vi "TiePie.Gen.Configure.vi"(8 "error in (no error)":errorcluster, 10 "Config":T1={"signal type (sine)"=1, "frequency"=0.0, "amplitude"=0.0, "offset"=0.0, "Enable"=FALSE} {"signal type (sine)" items=["sine"=1, "triangle"=2, "square"=4, "DC"=8, "noise"=16, "arbitrary"=32, "pulse"=64]}, 11 "GenHandle":T2) -> (0 "error out":errorcluster, 3 "GenHandle out":T2)   [LabVIEW 2013, in "LVTiePie.lvlib"]
uses:
  LVTiePie.lvlib
  TiePie.Gen.handle.ctl
  TiePie.Gen.CfgData.ctl
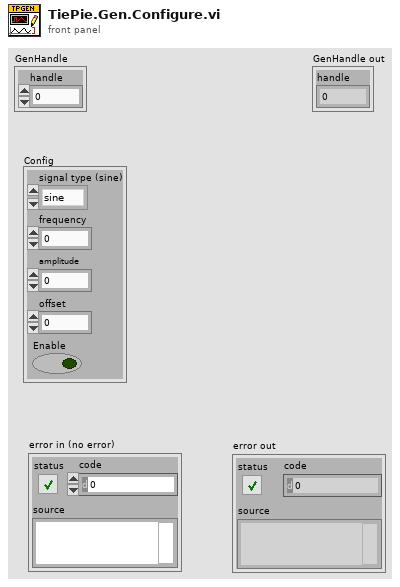
[diagram p1: front panel]
types:
  T1 = typedef "TiePie.Gen.CfgData.ctl" = cluster{"signal type (sine)":u32, "frequency":dbl, "amplitude":dbl, "offset":dbl, "Enable":bool}
  T2 = typedef "TiePie.Gen.handle.ctl" = cluster{"handle":u32}
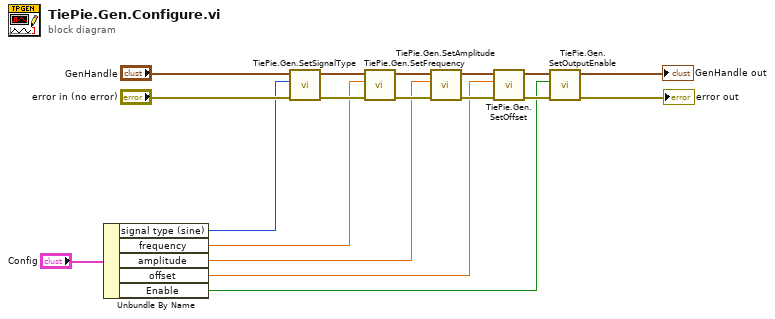
[diagram p0: block diagram]
diagram:
  n1 = Unbundle By Name("Config") -> ("signal type (sine)"=w5:u32, "frequency"=w4:dbl, "amplitude"=w3:dbl, "offset"=w2:dbl, "Enable"=w1:bool)
  n2 = call "TiePie.Gen.SetSignalType.vi"("error in (no error)"="error in (no error)", "signal type (sine)"=w5, "GenHandle"="GenHandle") -> ("error out"=w17:errorcluster, "GenHandle out"=w10:T2)  [unwired: 7 in]
  n3 = call "TiePie.Gen.SetFrequency.vi"("error in (no error)"=w17, "frequency"=w4, "GenHandle"=w10) -> ("error out"=w16:errorcluster, "GenHandle out"=w9:T2)  [unwired: 7 in]
  n4 = call "TiePie.Gen.SetAmplitude.vi"("error in (no error)"=w16, "amplitude"=w3, "GenHandle"=w9) -> ("error out"=w15:errorcluster, "GenHandle out"=w8:T2)  [unwired: 7 in]
  n5 = call "TiePie.Gen.SetOffset.vi"("error in (no error)"=w15, "offset"=w2, "GenHandle"=w8) -> ("error out"=w14:errorcluster, "GenHandle out"=w7:T2)  [unwired: 7 in]
  n6 = call "TiePie.Gen.SetOutputEnable.vi"("error in (no error)"=w14, "Enable"=w1, "GenHandle"=w7) -> ("error out"=→"error out":errorcluster, "GenHandle out"=→"GenHandle out":T2)  [unwired: 7 in]
